vi "Pasco_Drive(2013).vi"(9 "Power":dbl, 10 "Current Angle":dbl, 11 "Desired Angle":dbl) -> (2 "Left Drive":dbl, 3 "Right Drive":dbl)   [LabVIEW 2011]
panel:
  out "turn right?":bool
  out "Delta Angle":dbl
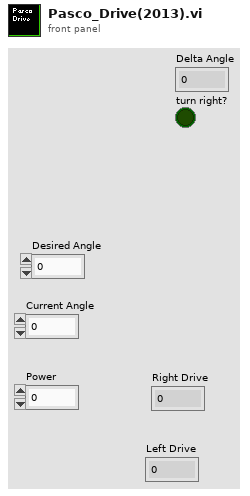
[diagram p1: front panel]
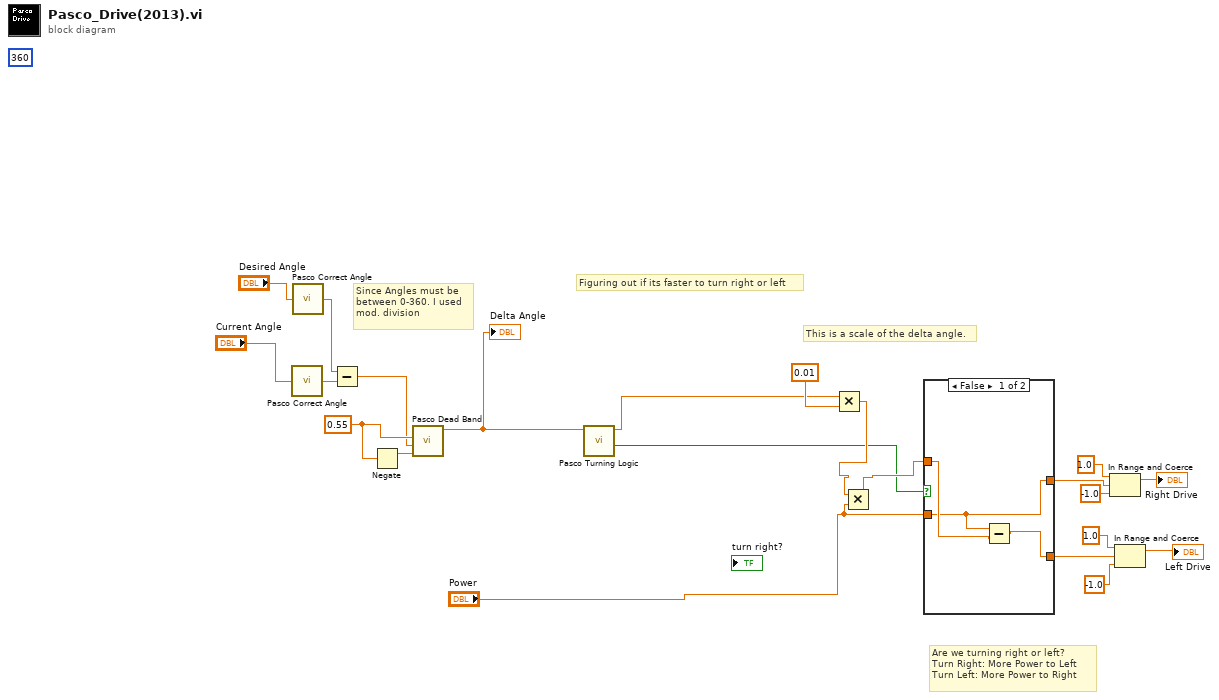
[diagram p0: block diagram]
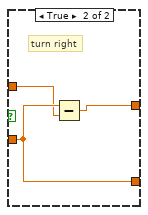
[diagram p2: hidden frame]
diagram:
  w21 = 0.55 ("upper limit")
  (unwired) 360
  # "Figuring out if its faster to turn right or left"
  # "Are we turning right or left?\nTurn Right: More Power to Left\nTurn Left: More Power to Right"
  # "This is a scale of the delta angle."
  # "Since Angles must be \nbetween 0-360. I used\nmod. division"
  n1 = call "Pasco Correct Angle.vi"("Given Angle"="Current Angle") -> ("Corrected Angle"=w10:dbl)
  n2 = call "Pasco Correct Angle.vi"("Given Angle"="Desired Angle") -> ("Corrected Angle"=w8:dbl)
  n3 = Subtract(x=w8, y=w10) -> (x-y=w20:dbl)
  n4 = Negate(x=w21) -> (-x=w22:dbl)
  n5 = call "Pasco Dead Band.vi"("lower limit"=w22, "PWM Power"=w20, "upper limit"=w21) -> ("PWM Power"=w3:dbl)  [unwired: 7 in, 1 out]
  "Delta Angle" <- w3
  n6 = call "Pasco Turning Logic.vi"("Delta Angle"=w3) -> ("Case Selector"=w1:bool, "Corrected Angle"=w2:dbl)  [unwired: 9 in]
  n7 = Multiply(x=w2, y=0.01) -> (x*y=w5:dbl)
  n8 = Multiply(x=w5, y="Power") -> (x*y=w6:dbl)
  n9 = case shown="False" w1 {
    tunnel: w6 -> [w24 w26]
    tunnel: "Power" -> [w23 w27]
    tunnel: [w23 w28] -> w12
    tunnel: [w25 w27] -> w11
    frame False {
      n10 = Subtract(x=w23, y=w24) -> (x-y=w25:dbl)
    }
    frame True {
      # "turn right"
      n11 = Subtract(x=w27, y=w26) -> (x-y=w28:dbl)
    }
  }
  n12 = In Range and Coerce(upper limit=1.0, x=w12, lower limit=-1.0) -> (coerced(x)=→"Right Drive":dbl)  [unwired: 1 out]
  n13 = In Range and Coerce(upper limit=1.0, x=w11, lower limit=-1.0) -> (coerced(x)=→"Left Drive":dbl)  [unwired: 1 out]
